vi "Plot attributes load new row.vi"(8 "error in (no error)":errorcluster, 10 "Plot Index":i32, 11 "Plot":refnum<vi>) -> (0 "error out":errorcluster, 3 "plot":refnum<vi>)   [LabVIEW 2021, in "RocketPlot.lvlib"]
uses:
  RocketPlot.lvlib
  <vilib>/Utility/colorconv.llb/RGB to Color.vi
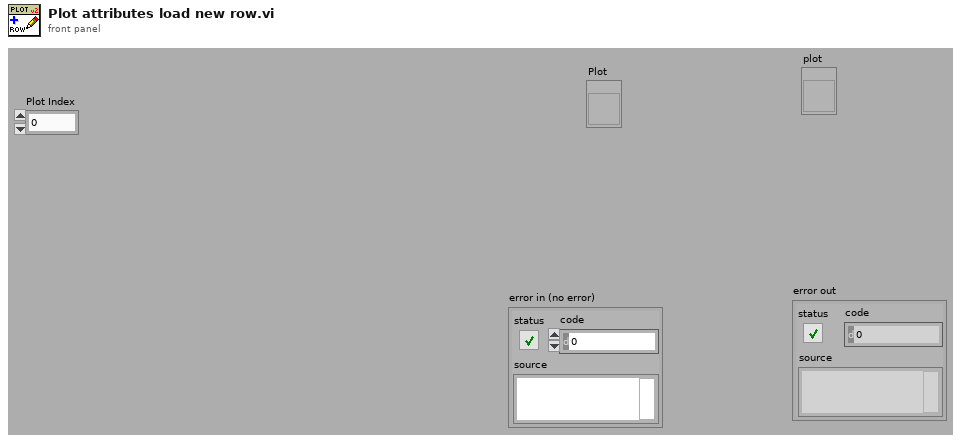
[diagram p1: front panel]
types:
  T1 = typedef "RocketPlot.lvlib/plot attributes V2.ctl" = cluster{"Plot Color":u32, "Point Style":u8, "Line Style":u8, "Plot Interpolation":u8, "Line Width":u8, "Bar Plot Style":u8, "Fill To":i16, "X Scale Index":u32, "Y Scale Index":u32, "Anti-aliased":bool, "Label Format":u8, "Digital Transition Type":u8, "Digital Transition Location":u8, "Digital Line Style":u8, "Fill/Point Color":u32, "Plot Name":string, "Visible":bool}
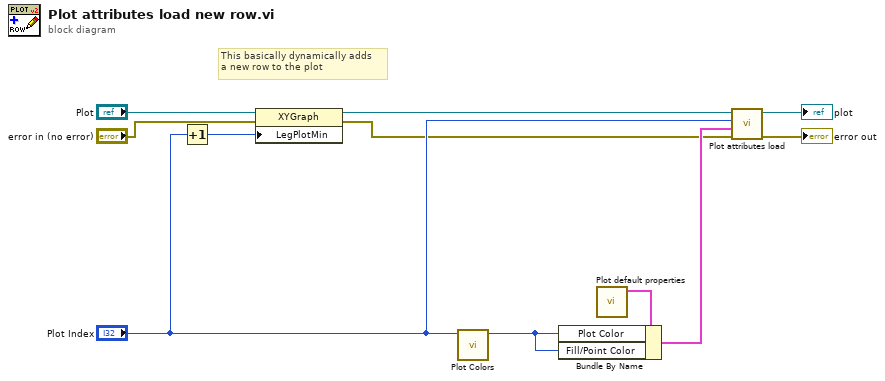
[diagram p0: block diagram]
diagram:
  # "This basically dynamically adds\na new row to the plot"
  n1 = Increment(x="Plot Index") -> (x+1=w4:i32)
  n2 = property class="XYGraph"(reference="Plot", error in="error in (no error)", "LegPlotMin"=w4) -> (reference out=w3:refnum<vi>, error out=w2:errorcluster)
  n3 = call "Plot Colors.vi"("Plot Index"="Plot Index") -> ("Color Box"=w11:u32)  [unwired: 10 in]
  n4 = call "Plot default properties.vi"() -> ("Default Attributes"=w1:T1)  [unwired: 7 in, 4 out]
  n5 = Bundle By Name(cluster=w1, "Plot Color"=w11, "Fill/Point Color"=w11) -> (w10:T1)
  n6 = call "Plot attributes load.vi"("error in (no error)"=w2, "attributes"=w10, "Active Plot"="Plot Index", "Plot"=w3) -> ("error out"=→"error out":errorcluster, "plot"=→"plot":refnum<vi>)  [unwired: 6 in]
